vi "FT_Get_Modem_Status.vi"(0 "Handle":u32) -> (1 "FT_Status":u32(ring) items=["FT_OK", "FT_INVALID_HANDLE", "FT_DEVICE_NOT_FOUND", "FT_DEVICE_NOT_OPENED", "FT_IO_ERROR", "FT_INSUFFICIENT_RESOURCES", "FT_INVALID_PARAMETER", "FT_INVALID_BAUD_RATE", "FT_DEVICE_NOT_OPENED_FOR_ERASE", "FT_DEVICE_NOT_OPENED_FOR_WRITE", "FT_FAILED_TO_WRITE_DEVICE", "FT_EEPROM_READ_FAILED", "FT_EEPROM_WRITE_FAILED", "FT_EEPROM_ERASE_FAILED", "FT_EEPROM_NOT_PRESENT", "FT_EEPROM_NOT_PROGRAMMED", "FT_INVALID_ARGS", "FT_NOT_SUPPORTED", "FT_OTHER_ERROR"], 2 "Modem Status":T2, 3 "Line Status":T1)   [LabVIEW 2016]
uses:
  FTD2XX.dll
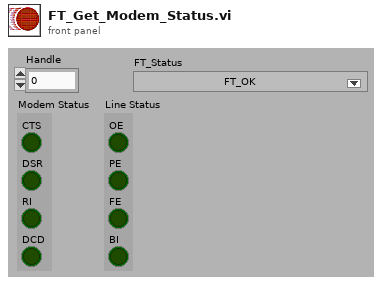
[diagram p1: front panel]
types:
  T1 = cluster{"OE":bool, "PE":bool, "FE":bool, "BI":bool}
  T2 = cluster{"CTS":bool, "DSR":bool, "RI":bool, "DCD":bool}
  T3 = cluster{"Boolean array[0]":bool, "Boolean array[1]":bool, "Boolean array[2]":bool, "Boolean array[3]":bool, "Boolean array[4]":bool, "Boolean array[5]":bool, "Boolean array[6]":bool, "Boolean array[7]":bool}
  T4 = cluster{"Boolean array[4]":bool, "Boolean array[5]":bool, "Boolean array[6]":bool, "Boolean array[7]":bool}
  T5 = cluster{"Boolean array[1]":bool, "Boolean array[2]":bool, "Boolean array[3]":bool, "Boolean array[4]":bool}
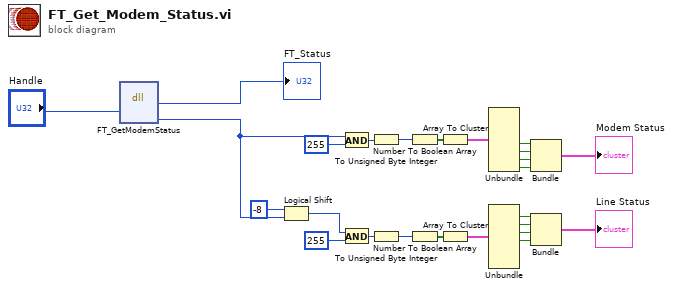
[diagram p0: block diagram]
diagram:
  n1 = dll-call lib="FTD2XX.dll" fn="FT_GetModemStatus"("Handle"="Handle") -> ("FT_Status"=→"FT_Status":u32, "ModemStatus"=w12:u32)  [unwired: 5 in, 2 out]
  n2 = Logical Shift(y=-8, x=w12) -> (x << y=w10:u32)
  n3 = And(x=w12, y=u32 255) -> (x .and. y?=w22:u32)
  n4 = And(x=w10, y=u32 255) -> (x .and. y?=w6:u32)
  n5 = To Unsigned Byte Integer(number=w22) -> (unsigned 8bit integer=w19:u8)
  n6 = To Unsigned Byte Integer(number=w6) -> (unsigned 8bit integer=w7:u8)
  n7 = Number To Boolean Array(number=w19) -> (Boolean array=w21:bool[])
  n8 = Number To Boolean Array(number=w7) -> (Boolean array=w9:bool[])
  n9 = Array To Cluster(array=w21) -> (cluster=w20:T3)
  n10 = Array To Cluster(array=w9) -> (cluster=w8:T3)
  n11 = Unbundle(w20) -> ("Boolean array[4]"=w14:bool, "Boolean array[5]"=w15:bool, "Boolean array[6]"=w16:bool, "Boolean array[7]"=w17:bool)  [unwired: 4 out]
  n12 = Unbundle(w8) -> ("Boolean array[1]"=w5:bool, "Boolean array[2]"=w4:bool, "Boolean array[3]"=w3:bool, "Boolean array[4]"=w2:bool)  [unwired: 4 out]
  n13 = Bundle("Boolean array[4]"=w14, "Boolean array[5]"=w15, "Boolean array[6]"=w16, "Boolean array[7]"=w17) -> (→"Modem Status":T4)  [unwired: 1 in]
  n14 = Bundle("Boolean array[1]"=w5, "Boolean array[2]"=w4, "Boolean array[3]"=w3, "Boolean array[4]"=w2) -> (→"Line Status":T5)  [unwired: 1 in]
